vi "Pod Code.vi"() -> ()   [LabVIEW 2017]
uses:
  Type Defs/Relays.ctl
  Type Defs/tempReadings.ctl
  Sensors/Power Sensor - Adafruit INA219/INA219 Measurements.ctl
  Type Defs/telemetryReading.ctl
  <vilib>/Utility/RT CPU Load.ctl
  Type Defs/PodState.ctl
  Type Defs/tofReading.ctl
  Type Defs/pressureReading.ctl
  Type Defs/allLaserReadings.ctl
  Type Defs/laserReading.ctl
  Type Defs/AnalogPressureReading.ctl
  Type Defs/criticalTelemetry.ctl
  Sensors/Time of Flight - VL6180/VL6180 Resource.ctl
  Sensors/Power Sensor - Adafruit INA219/INA219 Config Options.ctl
  Type Defs/thermopileSettings.ctl
  Sensors/Pressure Sensor - BMP180/BMP180 Config Options.ctl
  Type Defs/SensorStates.ctl
  Type Defs/allData.ctl
  <vilib>/Platform/TimedLoop/XDataNode/timing_clust.ctl
  <vilib>/Platform/TimedLoop/XDataNode/nitl_modes.ctl
  <vilib>/Platform/TimedLoop/XDataNode/wakeup.ctl
  <vilib>/myRIO/Instrument Drivers/Onboard IO/DIO/typedefs/DIO Reference.ctl
  <vilib>/myRIO/Common/Instrument Driver Framework/Utilities/typedefs/myRIO Generic Hardware Reference.ctl
  <vilib>/myRIO/Common/Instrument Driver Framework/Utilities/typedefs/Hardware Version Enum.ctl
  <vilib>/myRIO/Common/Instrument Driver Framework/Utilities/typedefs/myRIO v1.0 Reference.ctl
  <vilib>/myRIO/Common/Instrument Driver Framework/Utilities/typedefs/Generic FPGA Reference.ctl
  <vilib>/myRIO/Common/Instrument Driver Framework/myRIO v1.0/DIO/typedefs/DIO Channels List.ctl
  <vilib>/myRIO/Common/Instrument Driver Framework/myRIO v1.0/DIO/typedefs/DIO Channels Enum.ctl
  <vilib>/userdefined/High Color/nirio_resource_hc.ctl
  <vilib>/myRIO/Common/Instrument Driver Framework/Utilities/vis/Is FPGA Ref Available.vi
  <vilib>/myRIO/Common/Instrument Driver Framework/myRIO v1.0/DIO/vis/myRIO v1.1 Open DIO.vi
  <vilib>/myRIO/Instrument Drivers/Onboard IO/DIO/vis/Read.vi
  <vilib>/myRIO/Instrument Drivers/Onboard IO/DIO/vis/Write.vi
  <vilib>/myRIO/Common/Instrument Driver Framework/Utilities/vis/Validate Channels.vi
  <vilib>/myRIO/Common/Instrument Driver Framework/myRIO v1.0/DIO/vis/myRIO v1.0 Reserve DIO.vi
  <vilib>/myRIO/Common/Instrument Driver Framework/myRIO v1.0/Resource Manager/vis/myRIO v1.0 Reserve Channel List.vi
  <vilib>/myRIO/Common/Instrument Driver Framework/myRIO v1.0/DIO/vis/myRIO v1.0 Build MUX Configuration DIO.vi
  <vilib>/myRIO/Common/Instrument Driver Framework/myRIO v1.0/Resource Manager/vis/myRIO v1.0 Reserve Channel.vi
  <vilib>/myRIO/Common/Instrument Driver Framework/myRIO v1.0/Resource Manager/vis/myRIO v1.0 Unreserve Channel.vi
  <vilib>/myRIO/Common/Instrument Driver Framework/myRIO v1.0/Resource Manager/vis/myRIO v1.0 Create Configuration List.vi
  <vilib>/myRIO/Common/Instrument Driver Framework/myRIO v1.0/Resource Manager/vis/myRIO v1.0 Build Mutex Name.vi
  <vilib>/Utility/VariantDataType/GetNumericInfo.vi
  <vilib>/Utility/error.llb/Error Cluster From Error Code.vi
  <vilib>/myRIO/Common/Instrument Driver Framework/myRIO v1.0/myRIO v1.1 Open.vi
  <vilib>/myRIO/Common/Instrument Driver Framework/Utilities/vis/IO Manager.vi
  <vilib>/myRIO/Common/Instrument Driver Framework/Utilities/vis/Configuration Manager.vi
  <vilib>/myRIO/Common/Instrument Driver Framework/myRIO v1.0/Resource Manager/vis/myRIO v1.0 Configure IO.vi
  <vilib>/myRIO/Common/Instrument Driver Framework/myRIO v1.0/myRIO v1.0 Close.vi
  <vilib>/myRIO/Common/Instrument Driver Framework/myRIO v1.0/DIO/vis/myRIO v1.0 Write DIO.vi
  <vilib>/myRIO/Common/Instrument Driver Framework/myRIO v1.0/DIO/vis/myRIO v1.0 Read DIO.vi
  <vilib>/myRIO/Express VI/Onboard IO/DO/DO Express VI.xnode
  <vilib>/myRIO/Instrument Drivers/Onboard IO/DIO/vis/myRIO DIO Open.xnode
  <vilib>/platform/TimedLoop/XDataNode/XDataNode.xnode
  <vilib>/myRIO/Express VI/Onboard IO/DI/DI Express VI.xnode
  <vilib>/myRIO/Instrument Drivers/Onboard IO/DIO/DIO.lvlib
  <vilib>/Platform/TimedLoop/XDataNode/XDNodeRunTimeDep.lvlib
  <vilib>/NI_Real-Time Target Support.lvlib
panel:
  in  "Prior Lows":u8=10
  out "Data Snap Period":u32
  out "Slow Sensor Period":u32
  out "State Machine Period":u32
  out "Fast Sensor Period":u32
  out "Actuators":u32
  out "Latest Critical Telemetry":T1
  out "Analog Pressure Reading":T3
  out "Laser Error":errorcluster
  out "Laser Readings":T4
  out "Pressure Reading":T6
  out "ToF Readings":T7[](array[typedef])
  out "Pod State Status":T2
  in  "Logging":bool
  out "Sensor Error 2":errorcluster
  out "# elements in queue":i32
  out "CPU loads":T8[](array[typedef]) {"ISR (%)" format="%#.2f"; "Idle (%)" format="%#.2f"; "Background (%)" format="%#.2f"; "Normal (%)" format="%#.2f"; "Above Normal (%)" format="%#.2f"; "High (%)" format="%#.2g"; "Timed Structures (%)" format="%#.2g"; "Time Critical (%)" format="%#.2g"; "Total (%)" format="%#.2g"}
  out "Log":T9[][](array[typedef])
  in  "Power I2C Addrs":u8[](array[numeric])=[68, 65, 69] format="%.0x"
  out "Power Readings":T10[](array[typedef]) {"Current" format="%#.3g A"; "Power" format="%#.3g W"; "Shunt Voltage" format=" %#.3g V"; "Bus Voltage" format="%#.3g V"; "Voltage (Total)" format="%#.3g V"}
  out "ThermalReadings":T11[](array[typedef]) {"Ambient Temp (°F)" format="%.2f °F"; "Ambient Temp (°C)" format="%.2f °C"; "Object Temp (°F)" format="%.2f °F"; "Object Temp (°C)" format="%.2f °C"}
  in  "Thermal I2C Addrs":u8[](array[numeric])=[64, 67] format="%.0x"
  in  "Reset Count":bool
  in  "ToFs in use":T12[](array[typedef])=[enum."ToF1", enum."ToF2", enum."ToF3", enum."ToF4"]
  out "Sensor Error":errorcluster
  in  "Reset Sensors":bool
  out "State Error":errorcluster
  in  "Stop Button":bool
  # "Config"
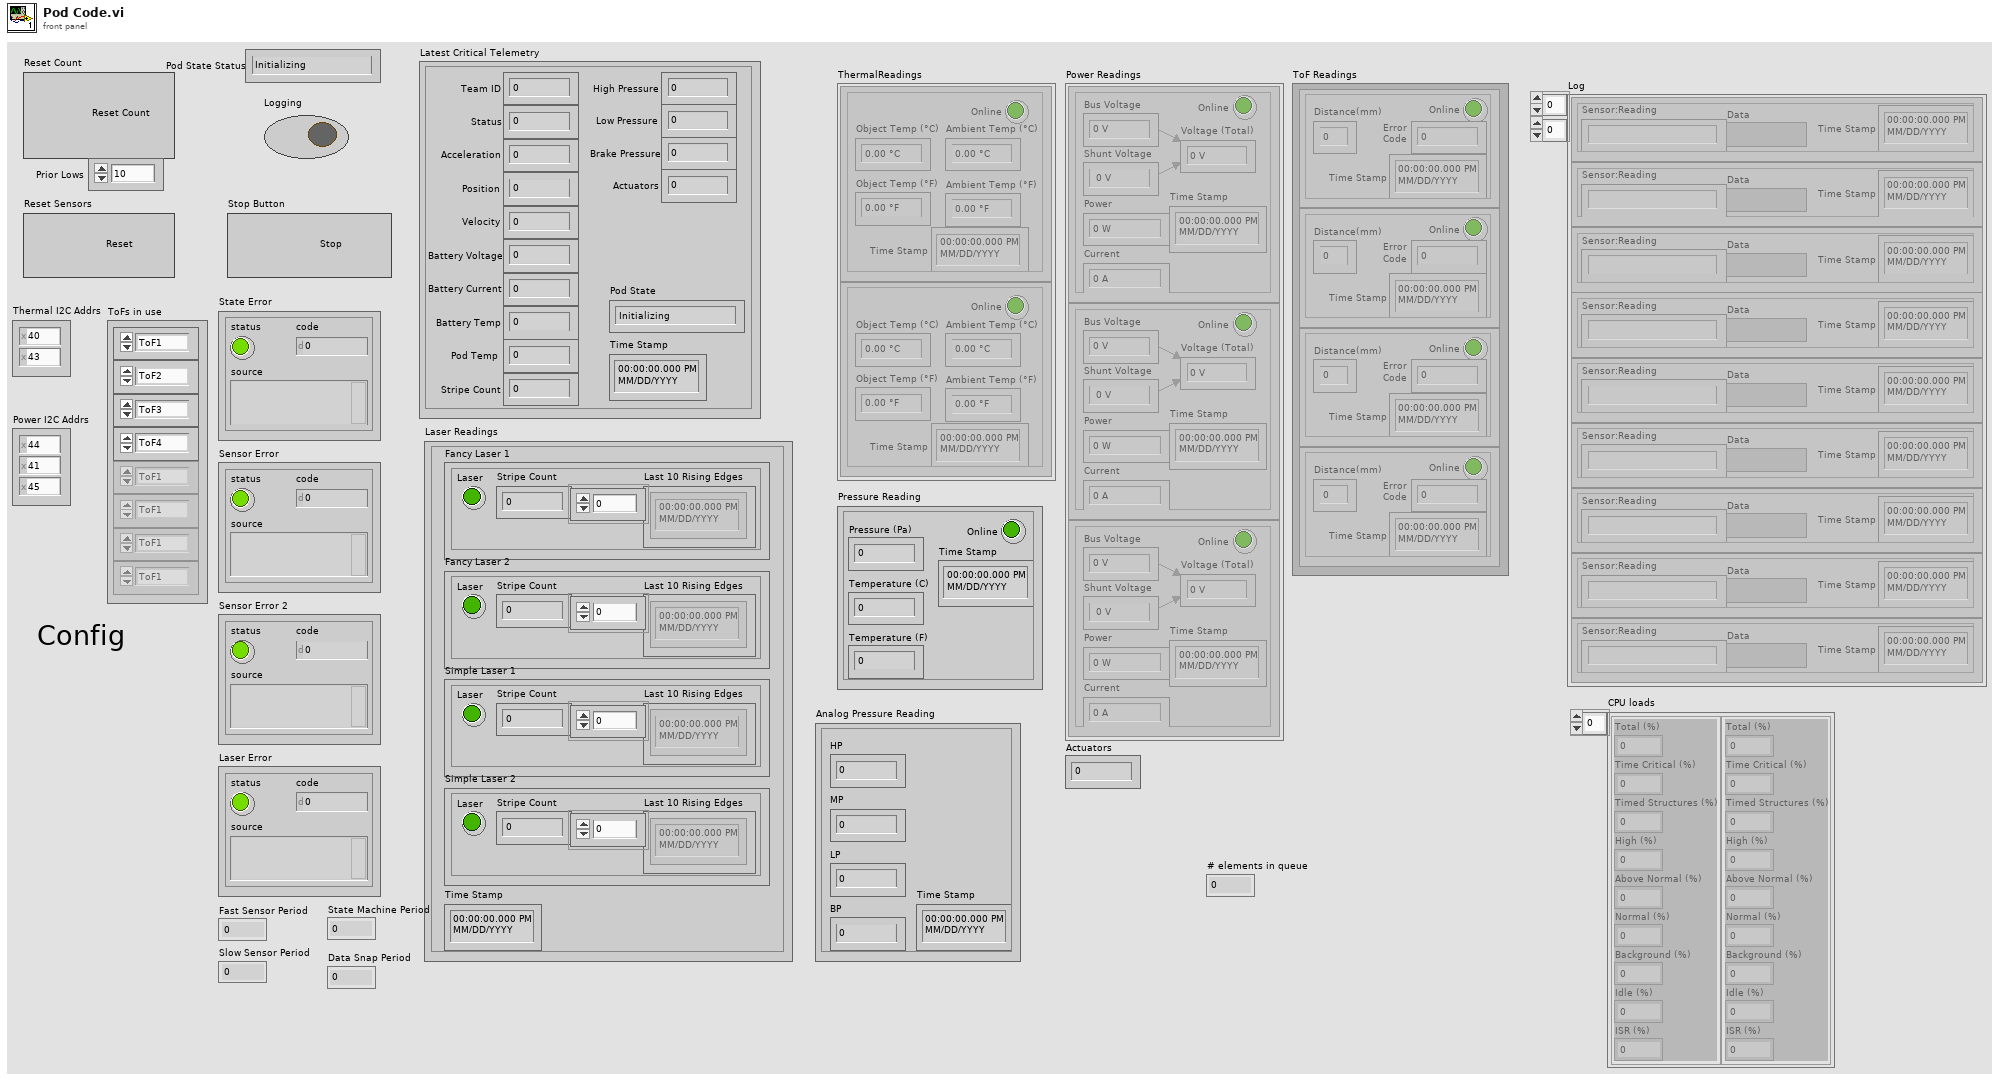
[diagram p1: front panel]
types:
  T1 = typedef "criticalTelemetry.ctl" = cluster{"Team ID":u8, "Status":u8, "Acceleration":i32, "Position":i32, "Velocity":i32, "Battery Voltage":i32, "Battery Current":i32, "Battery Temp":i32, "Pod Temp":i32, "Stripe Count":u32, "High Pressure":dbl, "Low Pressure":dbl, "Brake Pressure":dbl, "Actuators":u32, "Pod State":T2, "Time Stamp":timestamp}
  T2 = typedef "PodState.ctl" = enum16{"Initializing", "Pre-flight Testing", "Ready", "Pushing", "Coast", "Braking", "Post-flight", "Fault"}
  T3 = typedef "AnalogPressureReading.ctl" = cluster{"HP":dbl, "MP":dbl, "LP":dbl, "BP":dbl, "Time Stamp":timestamp}
  T4 = typedef "allLaserReadings.ctl" = cluster{"Fancy Laser 1":T5, "Fancy Laser 2":T5, "Simple Laser 1":T5, "Simple Laser 2":T5, "Time Stamp":timestamp}
  T5 = typedef "laserReading.ctl" = cluster{"Laser":bool, "Stripe Count":u32, "Last 10 Rising Edges":timestamp[]}
  T6 = typedef "pressureReading.ctl" = cluster{"Time Stamp":timestamp, "Online":bool, "Temperature (C)":dbl, "Pressure (Pa)":dbl, "Temperature (F)":dbl}
  T7 = typedef "tofReading.ctl" = cluster{"Distance(mm)":u8, "Online":bool, "Error\nCode":u8, "Time Stamp":timestamp}
  T8 = typedef "NI_Real-Time Target Support.lvlib/RT CPU Load.ctl" = cluster{"Total (%)":dbl, "Time Critical (%)":dbl, "Timed Structures (%)":dbl, "High (%)":dbl, "Above Normal (%)":dbl, "Normal (%)":dbl, "Background (%)":dbl, "Idle (%)":dbl, "ISR (%)":dbl}
  T9 = typedef "telemetryReading.ctl" = cluster{"Sensor:Reading":string, "Data":variant, "Time Stamp":timestamp}
  T10 = typedef "INA219 Measurements.ctl" = cluster{"Voltage (Total)":dbl, "Bus Voltage":dbl, "Shunt Voltage":dbl, "Power":dbl, "Current":dbl, "Online":bool, "Time Stamp":timestamp}
  T11 = typedef "tempReadings.ctl" = cluster{"Object Temp (°C)":dbl, "Object Temp (°F)":dbl, "Ambient Temp (°C)":dbl, "Ambient Temp (°F)":dbl, "Online":bool, "Time Stamp":timestamp}
  T12 = typedef "Relays.ctl" = enum16{"ToF1", "ToF2", "ToF3", "ToF4", "ToF5", "ToF6", "ToF7", "ToF8", "SensePwr", "All"}
  T13 = typedef "SensorStates.ctl" = enum16{"Reset", "Read", "Close"}
  T14 = typedef "BMP180 Config Options.ctl" = cluster{"I2C":cluster{"Slave Address":u8, "Channel":u8}, "Mode":enum8{"Ultra Low Power", "Standard", "High Resolution", "Ultra High Resolution"}, "Cal Coefs":cluster{"AC1":cluster{"Addr:":u8, "Val:":u16}, "AC2":cluster{"Addr:":u8, "Val:":u16}, "AC3":cluster{"Addr:":u8, "Val:":u16}, "AC4":cluster{"Addr:":u8, "Val:":u16}, "AC5":cluster{"Addr:":u8, "Val:":u16}, "AC6":cluster{"Addr:":u8, "Val:":u16}, "B1":cluster{"Addr:":u8, "Val:":u16}, "B2":cluster{"Addr:":u8, "Val:":u16}, "MB":cluster{"Addr:":u8, "Val:":u16}, "MC":cluster{"Addr:":u8, "Val:":u16}, "MD":cluster{"Addr:":u8, "Val:":u16}}, "Online":bool}
  T15 = typedef "thermopileSettings.ctl" = cluster{"Online":bool, "I2C Channel":u8, "I2C Slave Address":u8, "Valid Sample":bool, "Samples to Average":u16, "Last Temp Readings":T11, "Last Reading Time":dbl, "Last Conv Time":dbl}
  T16 = typedef "INA219 Config Options.ctl" = cluster{"I2C":cluster{"Slave Address":u8, "Channel":u8}, "Reset bit":u8, "Bus Voltage Range":u8, "PGA/Shunt Voltage Gain":u8, "Bus Voltage ADC Settings":u8, "Shunt Voltage ADC Settings":u8, "Mode":u8, "Calibration Value":u16, "Online":bool, "Shunt Resistor":dbl}
  T17 = typedef "VL6180 Resource.ctl" = cluster{"I2C Channel":u8, "I2C Slave Address":u8, "Online":bool}
  T18 = typedef "XDNodeRunTimeDep.lvlib/timing_clust.ctl" = cluster{"Expected End [f-1]":u64, "Actual End [f-1]":u64, "Finished Late? [f-1]":bool, "Expected End [i-1]":u64, "Actual End [i-1]":u64, "Finished Late? [i-1]":bool, "Expected Start [i]":u64, "Actual Start [i]":u64, "Expected Start [f]":u64, "Actual Start [f]":u64, "Source Name":string, "Structure Name":string, "Period":i64, "Deadline":i64, "Offset":i64, "Start":i64, "Priority":i32, "Timeout":i32, "Mode":T19, "Wakeup Reason":T20, "Error":errorcluster, "Source Type":string, "Secondary Source Type":string, "Global End Time":u64, "Global Start Time":u64, "Frame Duration":u64, "Iteration Duration":u64, "Assigned CPU":i32, "I/O Scan Engine Mode":u32}
  T19 = typedef "XDNodeRunTimeDep.lvlib/nitl_modes.ctl" = enum32{"No Change", "Process missed periods, maintain original phase", "Discard missed periods, maintain original phase", "Process missed periods, ignore original phase", "Discard missed periods, ignore original phase"}
  T20 = typedef "XDNodeRunTimeDep.lvlib/wakeup.ctl" = enum32{"Normal", "Aborted", "Asynchronous wakeup", "Timing source error", "Timed loop error", "Timeout"}
  T21 = typedef "DIO.lvlib/DIO Reference.ctl" = cluster{"myRIO Reference":T22, "DIO Channels List":T26}
  T22 = typedef "myRIO Generic Hardware Reference.ctl" = cluster{"myRIO Model":T23, "myRIO Hardware Reference":T24}
  T23 = typedef "Hardware Version Enum.ctl" = enum16{"Unknown", "myRIO-1900", "myRIO-1950", "roboRIO", "NI ELVIS RIO CM"}
  T24 = typedef "myRIO v1.0 Reference.ctl" = cluster{"Generic FPGA Reference":T25, "Allow multiple opens":bool}
  T25 = typedef "Generic FPGA Reference.ctl" = refnum<k20>
  T26 = typedef "DIO Channels List.ctl" = T27[]
  T27 = typedef "DIO Channels Enum.ctl" = enum16{"Not Connected", "C/DIO0", "C/DIO1", "C/DIO2", "C/DIO3", "C/DIO4", "C/DIO5", "C/DIO6", "C/DIO7", "A/DIO0", "A/DIO1", "A/DIO2", "A/DIO3", "A/DIO4", "A/DIO5", "A/DIO6", "A/DIO7", "A/DIO8", "A/DIO9", "A/DIO10", "A/DIO11", "A/DIO12", "A/DIO13", "A/DIO14", "A/DIO15", "B/DIO0", "B/DIO1", "B/DIO2", "B/DIO3", "B/DIO4", "B/DIO5", "B/DIO6", "B/DIO7", "B/DIO8", "B/DIO9", "B/DIO10", "B/DIO11", "B/DIO12", "B/DIO13", "B/DIO14", "B/DIO15", "LED0", "LED1", "LED2", "LED3", "Button0", "DIO/DIO0", "DIO/DIO1", "DIO/DIO2", "DIO/DIO3", "DIO/DIO4", "DIO/DIO5", "DIO/DIO6", "DIO/DIO7", "DIO/DIO8", "DIO/DIO9", "SPI/CS0", "SPI/CS1", "SPI/CS2", "SPI/CS3", "LED RADIO (Green)", "LED RADIO (Red)", "LED COMM (Green)", "LED COMM (Red)", "LED MODE (Green)", "LED MODE (Red)"}
  T28 = typedef "nirio_resource_hc.ctl" = tag
  T29 = typedef "allData.ctl" = cluster{"Power Readings":T10[], "ThermalReadings":T11[], "Analog Pressure Reading":T3, "Laser Readings":T4, "Pod State":T2, "seconds since 1Jan1904":timestamp, "ToF Readings":T7[], "CPU loads":T8[], "Actuators":u32, "Pressure Reading":T6, "Laser Error":errorcluster, "Sensor Error":errorcluster, "Sensor Error 2":errorcluster, "State Error":errorcluster}
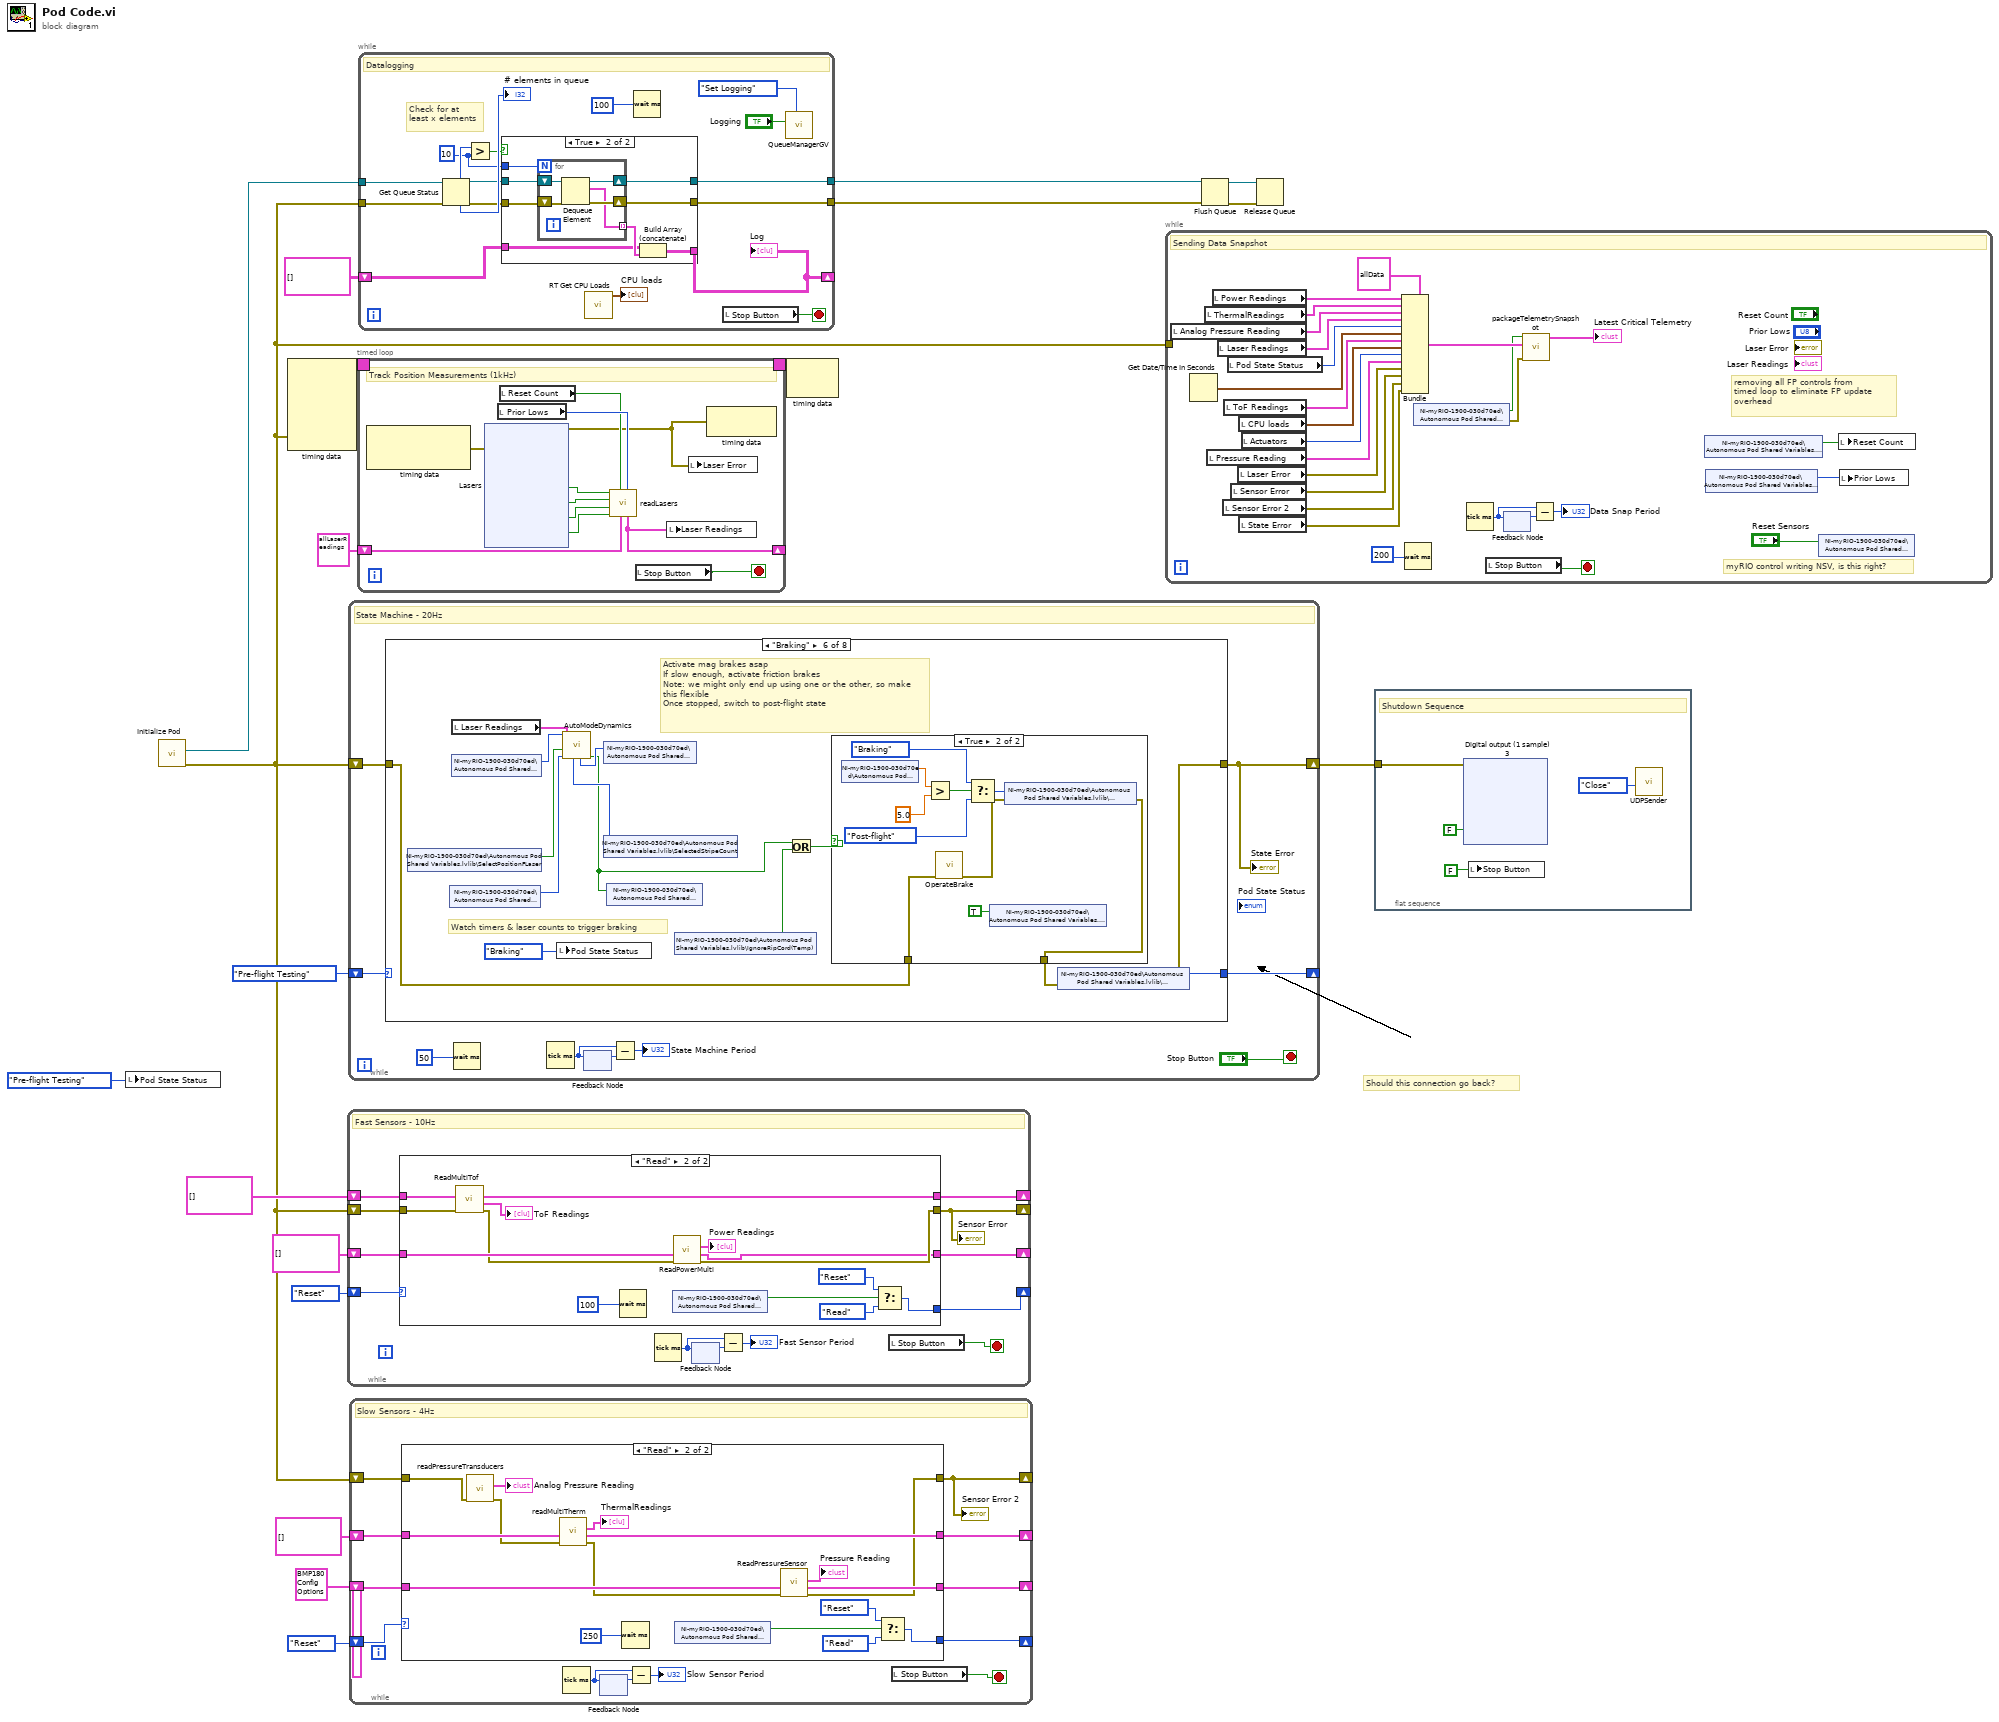
[diagram p0: block diagram]
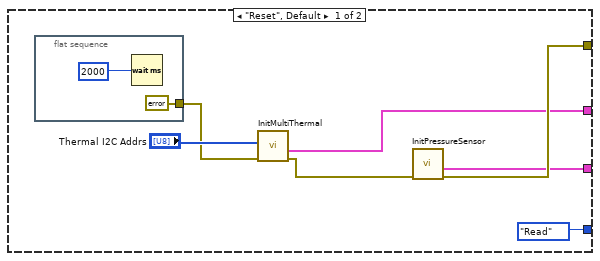
[diagram p3: hidden frame]
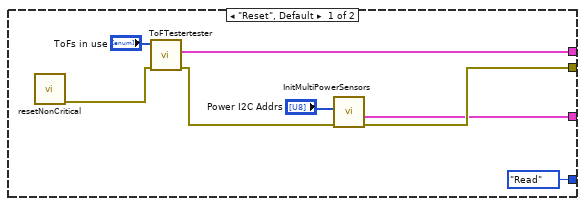
[diagram p4: hidden frame]
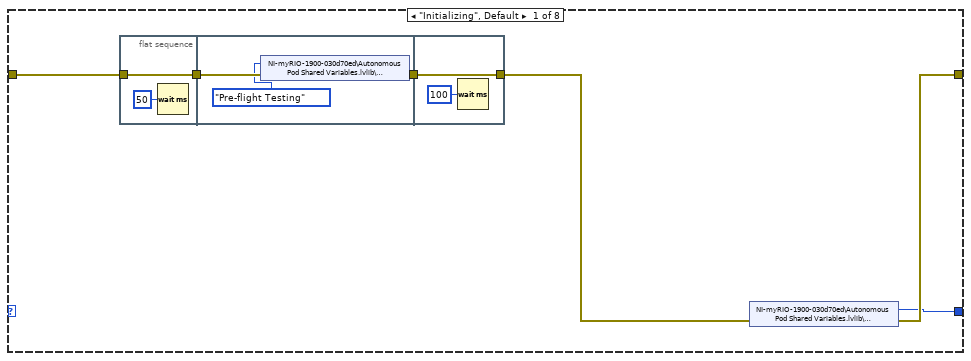
[diagram p5: hidden frame]
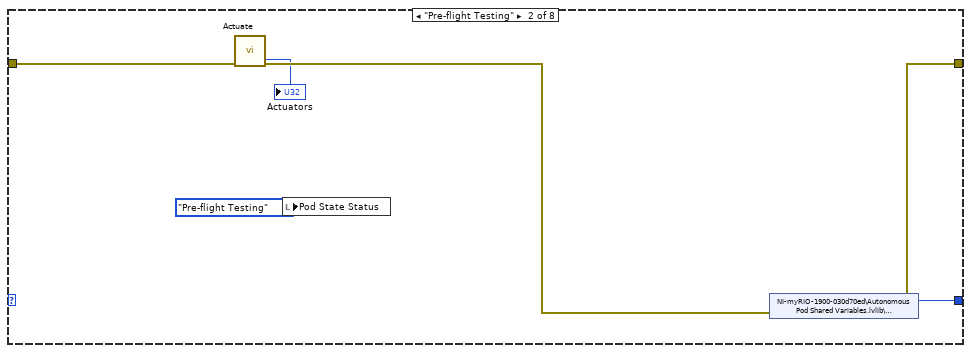
[diagram p6: hidden frame]
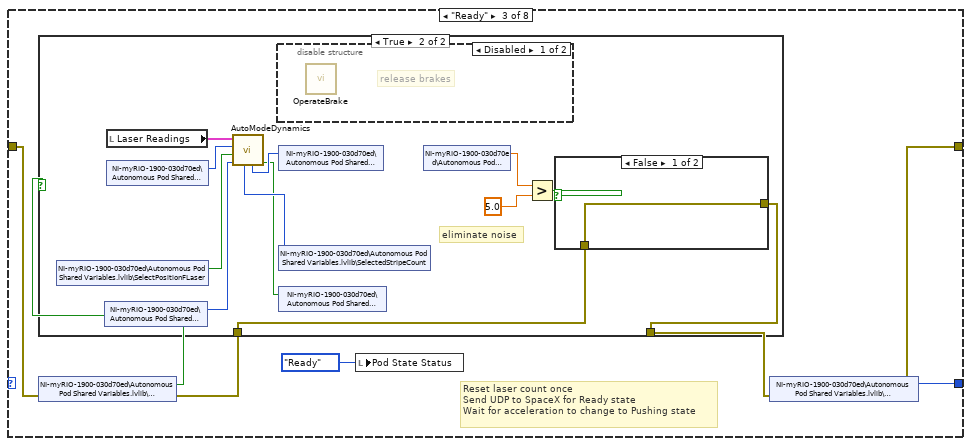
[diagram p7: hidden frame]
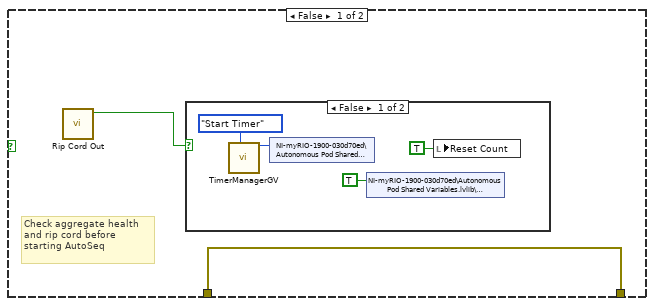
[diagram p8: hidden frame]
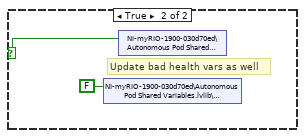
[diagram p9: hidden frame]
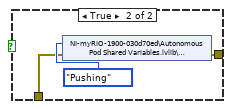
[diagram p11: hidden frame]
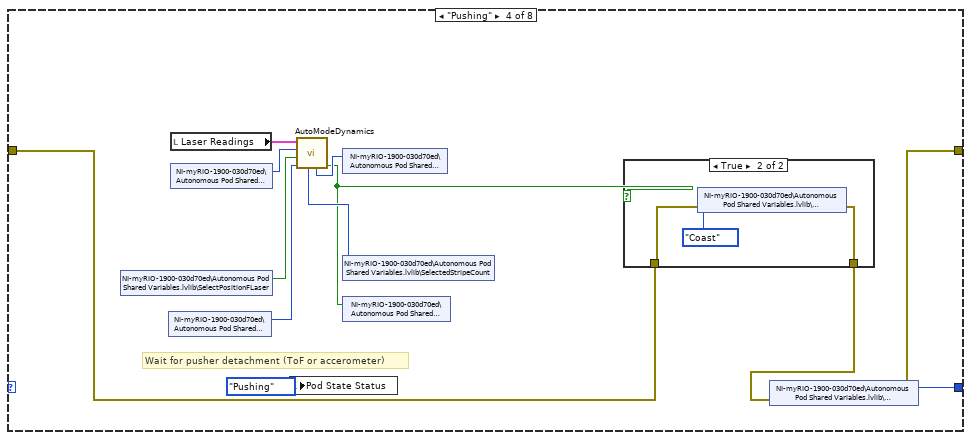
[diagram p12: hidden frame]
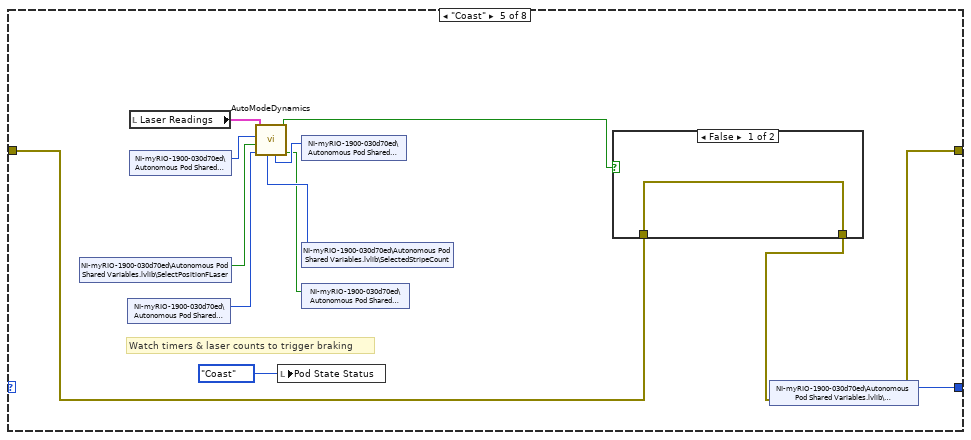
[diagram p14: hidden frame]
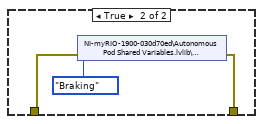
[diagram p15: hidden frame]
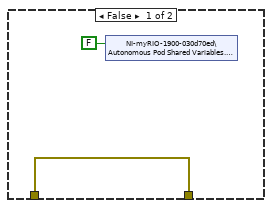
[diagram p16: hidden frame]
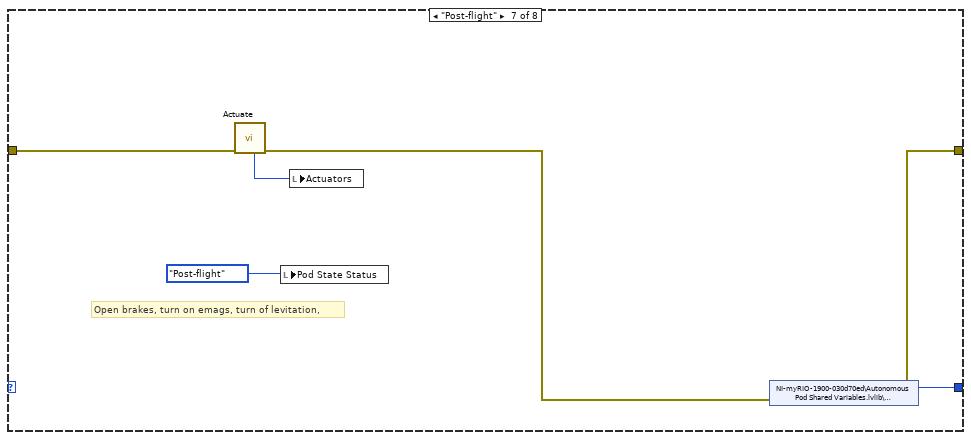
[diagram p17: hidden frame]
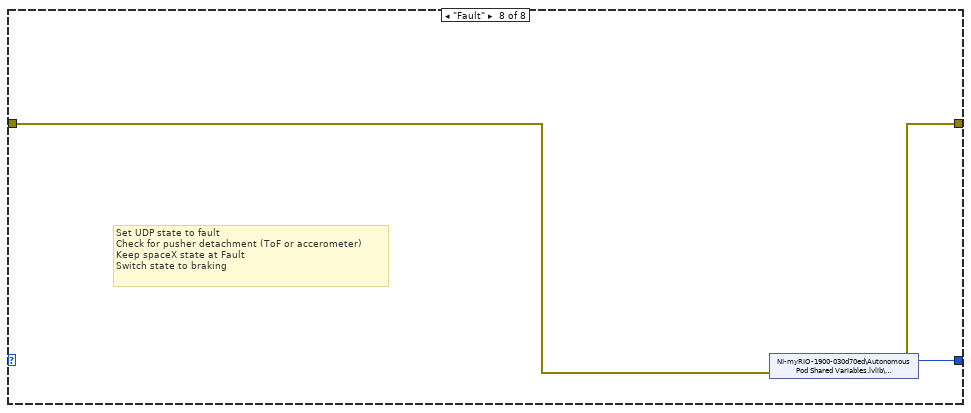
[diagram p18: hidden frame]
diagram:
  # "Should this connection go back?"
  n1 = local write "Pod State Status"(PodState."Pre-flight Testing" ("Pod State")) -> ()
  n2 = call "Initialize Pod.vi"() -> ("error out"=w3:errorcluster, "Telemetry Queue"=w16:refnum<queue>)  [unwired: 10 in]
  n3 = node-c288(w3) -> (w10:T18)  [unwired: 4 in]
  n4 = while {
    shift-right: [w29] -> _
    shift-left: SensorStates."Reset" -> [w31]
    shift-right: [w25] -> _
    shift-left: w3 -> [w30]
    shift-right: [w27] -> _
    shift-left: T17[] [] ("VL Configs") -> [w26]
    shift-right: [w20] -> _
    shift-left: T16[] [] ("Config Out") -> [w24]
    stop <- w28 stop-if-true
    # "Fast Sensors - 10Hz"
    n5 = case shown="\"Read\"" w31 {
      tunnel: w30 -> [_ w48]
      tunnel: [w35 w43] -> w25
      tunnel: [SensorStates."Read" w52] -> w29
      tunnel: [w32 w47] -> w27
      tunnel: w26 -> [_ w49]
      tunnel: w24 -> [_ w45]
      tunnel: [w33 w40] -> w20
      frame "Reset", Default {
        n6 = call "resetNonCritical.vi"() -> ("error out"=w38:errorcluster)  [unwired: 11 in]
        n7 = call "ToFTestertester.vi"("error in"=w38, "ToFs"="ToFs in use") -> ("error out"=w34:errorcluster, "ToF Details"=w32:T17[])  [unwired: 7 in, 1 out]
        n8 = call "InitMultiPowerSensors.vi"("error in"=w34, "I2C Addresses"="Power I2C Addrs") -> ("error out"=w35:errorcluster, "Power Sensors Configs"=w33:T16[])  [unwired: 7 in, 1 out]
      }
      frame "Read" {
        n9 = call "ReadMultiTof.vi"("error in"=w48, "VL6180 Resources"=w49) -> ("error out"=w42:errorcluster, "ToF Readings"=→"ToF Readings":T7[], "VL Configs"=w47:T17[])  [unwired: 6 in, 1 out]
        n10 = Wait (ms)(milliseconds to wait=u32 100) -> ()  [unwired: 1 out]
        n11 = shared-variable "NI-myRIO-1900-030d70ed\\Autonomous Pod Shared Variables.lvlib\\ResetSensor"() -> (w46:bool)  [unwired: 1 in, 1 out]
        n12 = call "ReadPowerMulti.vi"("error in"=w42, "Config In"=w45) -> ("error out"=w43:errorcluster, "Config Out"=w40:T16[], "Power Readings"=→"Power Readings":T10[])  [unwired: 7 in]
        n13 = Select(t=SensorStates."Reset", s=w46, f=SensorStates."Read") -> (s? t:f=w52:T13)
      }
    }
    "Sensor Error" <- w25
    n14 = Tick Count (ms)() -> (millisecond timer value=w22:u32)
    n15 = feedback-in #1(w22) -> ()
    n16 = feedback #1() -> (w23:u32)  [unwired: 1 in]
    n17 = Subtract(x=w22, y=w23) -> (x-y=→"Fast Sensor Period":u32)
    n18 = local read "Stop Button"() -> (w28:bool)
  }
  n19 = while {
    shift-right: [w58] -> w14
    shift-left: w3 -> [w60]
    shift-right: [w57] -> _
    shift-left: PodState."Pre-flight Testing" ("Pod States") -> [w59]
    stop <- "Stop Button" stop-if-true
    # "State Machine - 20Hz"
    n20 = case shown="\"Braking\"" w59 {
      tunnel: w60 -> [w68 w79 w85 w114 w131 w147 w175 w178]
      tunnel: [w64 w80 w87 w123 w140 w158 w176 w179] -> w58
      tunnel: [w63 w81 w88 w124 w141 w159 w177 w180] -> w57
      frame "Initializing", Default {
        n21 = flat-sequence {
          tunnel: w68 -> [w69]
          tunnel: [w69] -> w67
          tunnel: w67 -> [w73]
          tunnel: [w72] -> w65
          tunnel: [w74] -> w66
          tunnel: w65 -> [w74]
          frame #0 {
            n22 = Wait (ms)(milliseconds to wait=u32 50) -> ()  [unwired: 1 out]
          }
          frame #1 {
            n23 = shared-variable "NI-myRIO-1900-030d70ed\\Autonomous Pod Shared Variables.lvlib\\PodStateCommand"(PodState."Pre-flight Testing" ("Pod States"), error in=w73) -> (error out=w72:errorcluster)
          }
          frame #2 {
            n24 = Wait (ms)(milliseconds to wait=u32 100) -> ()  [unwired: 1 out]
          }
        }
        n25 = shared-variable "NI-myRIO-1900-030d70ed\\Autonomous Pod Shared Variables.lvlib\\PodStateCommand"(error in=w66) -> (w63:T2, error out=w64:errorcluster)
      }
      frame "Pre-flight Testing" {
        n26 = call "Actuate.vi"("error in"=w79) -> ("error out"=w78:errorcluster, "Actuators"=→"Actuators":u32)  [unwired: 8 in, 1 out]
        n27 = local write "Pod State Status"(PodState."Pre-flight Testing" ("Pod State")) -> ()
        n28 = shared-variable "NI-myRIO-1900-030d70ed\\Autonomous Pod Shared Variables.lvlib\\PodStateCommand"(error in=w78) -> (w81:T2, error out=w80:errorcluster)
      }
      frame "Ready" {
        # "Reset laser count once\nSend UDP to SpaceX for Ready state\nWait for acceleration to change to Pushing state"
        n29 = shared-variable "NI-myRIO-1900-030d70ed\\Autonomous Pod Shared Variables.lvlib\\AutoSequenceOn"(error in=w85) -> (w86:bool, error out=w83:errorcluster)
        n30 = case shown="True" w86 {
          tunnel: w83 -> [w89 w98]
          tunnel: [w89 w97] -> w82
          frame False {
            # "Check aggregate health and rip cord before starting AutoSeq"
            n31 = call "Rip Cord Out"() -> ("Rip Cord Out?"=w90:bool)  [unwired: 11 in]
            n32 = case shown="False" w90 {
              selector: w90 -> [_ w96]
              frame False {
                n33 = call "TimerManagerGV.vi"("Command"=enum16{"Get Time Elapsed", "Start Timer"}."Start Timer") -> ("Timer Value(s)"=w91:u32)  [unwired: 9 in, 1 out]
                n34 = shared-variable "NI-myRIO-1900-030d70ed\\Autonomous Pod Shared Variables.lvlib\\TimerValue"(w91) -> ()  [unwired: 1 in, 1 out]
                n35 = shared-variable "NI-myRIO-1900-030d70ed\\Autonomous Pod Shared Variables.lvlib\\AutoSequenceOn"(TRUE ("AutoSequenceOn")) -> ()  [unwired: 1 in, 1 out]
                n36 = local write "Reset Count"(TRUE ("Reset Count")) -> ()
              }
              frame True {
                # "Update bad health vars as well"
                n37 = shared-variable "NI-myRIO-1900-030d70ed\\Autonomous Pod Shared Variables.lvlib\\AutoSequenceOn"(FALSE ("AutoSequenceOn")) -> ()  [unwired: 1 in, 1 out]
                n38 = shared-variable "NI-myRIO-1900-030d70ed\\Autonomous Pod Shared Variables.lvlib\\RipCordOut"(w96) -> ()  [unwired: 1 in, 1 out]
              }
            }
          }
          frame True {
            # "eliminate noise"
            n39 = shared-variable "NI-myRIO-1900-030d70ed\\Autonomous Pod Shared Variables.lvlib\\SelectPositionFLaser"() -> (w106:bool)  [unwired: 1 in, 1 out]
            n40 = shared-variable "NI-myRIO-1900-030d70ed\\Autonomous Pod Shared Variables.lvlib\\TimerLimit"() -> (w105:u32)  [unwired: 1 in, 1 out]
            n41 = local read "Laser Readings"() -> (w107:T4)
            n42 = shared-variable "NI-myRIO-1900-030d70ed\\Autonomous Pod Shared Variables.lvlib\\StripeLimit"() -> (w108:u32)  [unwired: 1 in, 1 out]
            n43 = call "AutoModeDynamics.vi"("Timer Limit"=w105, "SelectFLaser"=w106, "Stripe Limit"=w108, "Laser Readings"=w107) -> ("Rip Cord Out?"=w102:bool, "Timer Value(s)"=w104:u32, "Stripe Count"=w103:u32)  [unwired: 2 in, 3 out]
            n44 = disable-structure shown="Disabled" {
              frame Disabled {
                # "release brakes"
                n45 = call "OperateBrake.vi"() -> ()  [unwired: 11 in, 1 out]
              }
              frame Enabled {
              }
            }
            n46 = shared-variable "NI-myRIO-1900-030d70ed\\Autonomous Pod Shared Variables.lvlib\\TimerValue"(w104) -> ()  [unwired: 1 in, 1 out]
            n47 = shared-variable "NI-myRIO-1900-030d70ed\\Autonomous Pod Shared Variables.lvlib\\SelectedStripeCount"(w103) -> ()  [unwired: 1 in, 1 out]
            n48 = shared-variable "NI-myRIO-1900-030d70ed\\Autonomous Pod Shared Variables.lvlib\\RipCordOut"(w102) -> ()  [unwired: 1 in, 1 out]
            n49 = shared-variable "NI-myRIO-1900-030d70ed\\Autonomous Pod Shared Variables.lvlib\\Velocity"() -> (w101:dbl)  [unwired: 1 in, 1 out]
            n50 = Greater?(x=w101, y=5.0) -> (0:w99:bool)
            n51 = case shown="False" w99 {
              tunnel: w98 -> [w109 w111]
              tunnel: [w109 w110] -> w97
              frame False {
              }
              frame True {
                n52 = shared-variable "NI-myRIO-1900-030d70ed\\Autonomous Pod Shared Variables.lvlib\\PodStateCommand"(PodState."Pushing" ("Pod States"), error in=w111) -> (error out=w110:errorcluster)
              }
            }
          }
        }
        n53 = local write "Pod State Status"(PodState."Ready" ("Pod State")) -> ()
        n54 = shared-variable "NI-myRIO-1900-030d70ed\\Autonomous Pod Shared Variables.lvlib\\PodStateCommand"(error in=w82) -> (w88:T2, error out=w87:errorcluster)
      }
      frame "Pushing" {
        # "Wait for pusher detachment (ToF or accerometer)"
        n55 = shared-variable "NI-myRIO-1900-030d70ed\\Autonomous Pod Shared Variables.lvlib\\SelectPositionFLaser"() -> (w119:bool)  [unwired: 1 in, 1 out]
        n56 = shared-variable "NI-myRIO-1900-030d70ed\\Autonomous Pod Shared Variables.lvlib\\TimerLimit"() -> (w118:u32)  [unwired: 1 in, 1 out]
        n57 = local read "Laser Readings"() -> (w120:T4)
        n58 = shared-variable "NI-myRIO-1900-030d70ed\\Autonomous Pod Shared Variables.lvlib\\StripeLimit"() -> (w121:u32)  [unwired: 1 in, 1 out]
        n59 = local write "Pod State Status"(PodState."Pushing" ("Pod State")) -> ()
        n60 = call "AutoModeDynamics.vi"("Timer Limit"=w118, "SelectFLaser"=w119, "Stripe Limit"=w121, "Laser Readings"=w120) -> ("Rip Cord Out?"=w115:bool, "Timer Value(s)"=w117:u32, "Stripe Count"=w116:u32)  [unwired: 2 in, 3 out]
        n61 = shared-variable "NI-myRIO-1900-030d70ed\\Autonomous Pod Shared Variables.lvlib\\TimerValue"(w117) -> ()  [unwired: 1 in, 1 out]
        n62 = shared-variable "NI-myRIO-1900-030d70ed\\Autonomous Pod Shared Variables.lvlib\\SelectedStripeCount"(w116) -> ()  [unwired: 1 in, 1 out]
        n63 = shared-variable "NI-myRIO-1900-030d70ed\\Autonomous Pod Shared Variables.lvlib\\RipCordOut"(w115) -> ()  [unwired: 1 in, 1 out]
        n64 = case shown="True" w115 {
          tunnel: w114 -> [w125 w127]
          tunnel: [w125 w126] -> w113
          frame False {
          }
          frame True {
            n65 = shared-variable "NI-myRIO-1900-030d70ed\\Autonomous Pod Shared Variables.lvlib\\PodStateCommand"(PodState."Coast" ("PodStateCommand"), error in=w127) -> (error out=w126:errorcluster)
          }
        }
        n66 = shared-variable "NI-myRIO-1900-030d70ed\\Autonomous Pod Shared Variables.lvlib\\PodStateCommand"(error in=w113) -> (w124:T2, error out=w123:errorcluster)
      }
      frame "Coast" {
        # "Watch timers & laser counts to trigger braking"
        n67 = shared-variable "NI-myRIO-1900-030d70ed\\Autonomous Pod Shared Variables.lvlib\\SelectPositionFLaser"() -> (w137:bool)  [unwired: 1 in, 1 out]
        n68 = shared-variable "NI-myRIO-1900-030d70ed\\Autonomous Pod Shared Variables.lvlib\\TimerLimit"() -> (w136:u32)  [unwired: 1 in, 1 out]
        n69 = local read "Laser Readings"() -> (w138:T4)
        n70 = shared-variable "NI-myRIO-1900-030d70ed\\Autonomous Pod Shared Variables.lvlib\\StripeLimit"() -> (w139:u32)  [unwired: 1 in, 1 out]
        n71 = call "AutoModeDynamics.vi"("Timer Limit"=w136, "SelectFLaser"=w137, "Stripe Limit"=w139, "Laser Readings"=w138) -> ("Rip Cord Out?"=w133:bool, "Brake Condition Reached?"=w129:bool, "Timer Value(s)"=w135:u32, "Stripe Count"=w134:u32)  [unwired: 2 in, 2 out]
        n72 = local write "Pod State Status"(PodState."Coast" ("Pod State")) -> ()
        n73 = shared-variable "NI-myRIO-1900-030d70ed\\Autonomous Pod Shared Variables.lvlib\\TimerValue"(w135) -> ()  [unwired: 1 in, 1 out]
        n74 = shared-variable "NI-myRIO-1900-030d70ed\\Autonomous Pod Shared Variables.lvlib\\SelectedStripeCount"(w134) -> ()  [unwired: 1 in, 1 out]
        n75 = shared-variable "NI-myRIO-1900-030d70ed\\Autonomous Pod Shared Variables.lvlib\\RipCordOut"(w133) -> ()  [unwired: 1 in, 1 out]
        n76 = case shown="False" w129 {
          tunnel: w131 -> [w142 w144]
          tunnel: [w142 w143] -> w130
          frame False {
          }
          frame True {
            n77 = shared-variable "NI-myRIO-1900-030d70ed\\Autonomous Pod Shared Variables.lvlib\\PodStateCommand"(PodState."Braking" ("PodStateCommand"), error in=w144) -> (error out=w143:errorcluster)
          }
        }
        n78 = shared-variable "NI-myRIO-1900-030d70ed\\Autonomous Pod Shared Variables.lvlib\\PodStateCommand"(error in=w130) -> (w141:T2, error out=w140:errorcluster)
      }
      frame "Braking" {
        # "Watch timers & laser counts to trigger braking"
        # "Activate mag brakes asap\nIf slow enough, activate friction brakes\nNote: we might only end up using one or the other, so make this flexible\nOnce stopped, switch to post-flight state"
        n79 = shared-variable "NI-myRIO-1900-030d70ed\\Autonomous Pod Shared Variables.lvlib\\SelectPositionFLaser"() -> (w155:bool)  [unwired: 1 in, 1 out]
        n80 = shared-variable "NI-myRIO-1900-030d70ed\\Autonomous Pod Shared Variables.lvlib\\TimerLimit"() -> (w154:u32)  [unwired: 1 in, 1 out]
        n81 = local read "Laser Readings"() -> (w156:T4)
        n82 = shared-variable "NI-myRIO-1900-030d70ed\\Autonomous Pod Shared Variables.lvlib\\StripeLimit"() -> (w157:u32)  [unwired: 1 in, 1 out]
        n83 = local write "Pod State Status"(PodState."Braking" ("Pod State")) -> ()
        n84 = call "AutoModeDynamics.vi"("Timer Limit"=w154, "SelectFLaser"=w155, "Stripe Limit"=w157, "Laser Readings"=w156) -> ("Rip Cord Out?"=w149:bool, "Timer Value(s)"=w153:u32, "Stripe Count"=w152:u32)  [unwired: 2 in, 3 out]
        n85 = shared-variable "NI-myRIO-1900-030d70ed\\Autonomous Pod Shared Variables.lvlib\\TimerValue"(w153) -> ()  [unwired: 1 in, 1 out]
        n86 = shared-variable "NI-myRIO-1900-030d70ed\\Autonomous Pod Shared Variables.lvlib\\SelectedStripeCount"(w152) -> ()  [unwired: 1 in, 1 out]
        n87 = shared-variable "NI-myRIO-1900-030d70ed\\Autonomous Pod Shared Variables.lvlib\\RipCordOut"(w149) -> ()  [unwired: 1 in, 1 out]
        n88 = shared-variable "NI-myRIO-1900-030d70ed\\Autonomous Pod Shared Variables.lvlib\\IgnoreRipCord(Temp)"() -> (w148:bool)  [unwired: 1 in, 1 out]
        n89 = Or(x=w149, y=w148) -> (x .or. y?=w150:bool)
        n90 = case shown="True" w150 {
          tunnel: [w161 w171] -> w146
          tunnel: w147 -> [w161 w163]
          frame False {
            n91 = shared-variable "NI-myRIO-1900-030d70ed\\Autonomous Pod Shared Variables.lvlib\\OperatingBrakes"(FALSE ("OperatingBrakes")) -> ()  [unwired: 1 in, 1 out]
          }
          frame True {
            n92 = shared-variable "NI-myRIO-1900-030d70ed\\Autonomous Pod Shared Variables.lvlib\\Velocity"() -> (w170:dbl)  [unwired: 1 in, 1 out]
            n93 = Greater?(x=w170, y=5.0) -> (0:w168:bool)
            n94 = call "OperateBrake.vi"("error in"=w163) -> ("error out"=w164:errorcluster)  [unwired: 10 in]
            n95 = Select(t=PodState."Braking" ("PodStateCommand"), s=w168, f=PodState."Post-flight" ("PodStateCommand")) -> (s? t:f=w166:T2)
            n96 = shared-variable "NI-myRIO-1900-030d70ed\\Autonomous Pod Shared Variables.lvlib\\OperatingBrakes"(TRUE ("OperatingBrakes")) -> ()  [unwired: 1 in, 1 out]
            n97 = shared-variable "NI-myRIO-1900-030d70ed\\Autonomous Pod Shared Variables.lvlib\\PodStateCommand"(w166, error in=w164) -> (error out=w171:errorcluster)
          }
        }
        n98 = shared-variable "NI-myRIO-1900-030d70ed\\Autonomous Pod Shared Variables.lvlib\\PodStateCommand"(error in=w146) -> (w159:T2, error out=w158:errorcluster)
      }
      frame "Post-flight" {
        # "Open brakes, turn on emags, turn of levitation,"
        n99 = call "Actuate.vi"("error in"=w175) -> ("error out"=w174:errorcluster, "Actuators"=w173:u32)  [unwired: 8 in, 1 out]
        n100 = local write "Pod State Status"(PodState."Post-flight" ("Pod State")) -> ()
        n101 = local write "Actuators"(w173) -> ()
        n102 = shared-variable "NI-myRIO-1900-030d70ed\\Autonomous Pod Shared Variables.lvlib\\PodStateCommand"(error in=w174) -> (w177:T2, error out=w176:errorcluster)
      }
      frame "Fault" {
        # "Set UDP state to fault\nCheck for pusher detachment (ToF or accerometer)\nKeep spaceX state at Fault\nSwitch state to braking"
        n103 = shared-variable "NI-myRIO-1900-030d70ed\\Autonomous Pod Shared Variables.lvlib\\PodStateCommand"(error in=w178) -> (w180:T2, error out=w179:errorcluster)
      }
    }
    "State Error" <- w58
    n104 = Wait (ms)(milliseconds to wait=u32 50) -> ()  [unwired: 1 out]
    n105 = Tick Count (ms)() -> (millisecond timer value=w54:u32)
    n106 = feedback #2() -> (w55:u32)  [unwired: 1 in]
    n107 = feedback-in #2(w54) -> ()
    n108 = Subtract(x=w54, y=w55) -> (x-y=→"State Machine Period":u32)
  }
  n109 = while {
    shift-right: [w190] -> _
    shift-left: SensorStates."Reset" -> [w192]
    shift-right: [w188] -> _
    shift-left: w3 -> [w191]
    shift-right: [w187] -> _
    shift-left: T15[] [] ("ThermalConfigs") -> [w186]
    shift-right: [w185] -> _
    shift-left: T14 {"I2C"={"Slave Address"=64, "Channel"=0}, "Mode"=enum."Ultra Low Power", "Cal Coefs"={"AC1"={"Addr:"=170, "Val:"=0}, "AC2"={"Addr:"=172, "Val:"=0}, "AC3"={"Addr:"=174, "Val:"=0}, "AC4"={"Addr:"=176, "Val:"=0}, "AC5"={"Addr:"=178, "Val:"=0}, "AC6"={"Addr:"=180, "Val:"=0}, "B1"={"Addr:"=182, "Val:"=0}, "B2"={"Addr:"=184, "Val:"=0}, "MB"={"Addr:"=186, "Val:"=0}, "MC"={"Addr:"=188, "Val:"=0}, "MD"={"Addr:"=190, "Val:"=0}}, "Online"=FALSE} ("BMP180 Config Options") -> [w184]
    stop <- w189 stop-if-true
    # "Slow Sensors - 4Hz"
    n110 = case shown="\"Read\"" w192 {
      tunnel: w191 -> [_ w205]
      tunnel: [w198 w208] -> w188
      tunnel: [SensorStates."Read" w216] -> w190
      tunnel: [w193 w212] -> w187
      tunnel: w186 -> [_ w211]
      tunnel: [w195 w209] -> w185
      tunnel: w184 -> [_ w210]
      frame "Reset", Default {
        n111 = flat-sequence {
          tunnel: [errorcluster {"status"=FALSE, "code"=0, "source"=""} ("error in")] -> w194
          frame #0 {
            n112 = Wait (ms)(milliseconds to wait=u32 2000) -> ()  [unwired: 1 out]
          }
        }
        n113 = call "InitMultiThermal.vi"("error in"=w194, "I2C Addresses"="Thermal I2C Addrs") -> ("error out"=w196:errorcluster, "ThermalConfigs"=w193:T15[])  [unwired: 6 in, 2 out]
        n114 = call "InitPressureSensor.vi"("error in"=w196) -> ("error out"=w198:errorcluster, "BMP180 Config Options"=w195:T14)  [unwired: 9 in]
      }
      frame "Read" {
        n115 = call "readPressureTransducers.vi"("error in"=w205) -> ("error out"=w204:errorcluster, "Analog Pressure Reading"=→"Analog Pressure Reading":T3)  [unwired: 9 in]
        n116 = call "readMultiTherm.vi"("error in"=w204, "ThermalConfigs"=w211) -> ("error out"=w206:errorcluster, "ThermalConfigs"=w212:T15[], "ThermReadings"=→"ThermalReadings":T11[])  [unwired: 6 in, 1 out]
        n117 = Wait (ms)(milliseconds to wait=u32 250) -> ()  [unwired: 1 out]
        n118 = shared-variable "NI-myRIO-1900-030d70ed\\Autonomous Pod Shared Variables.lvlib\\ResetSensor"() -> (w213:bool)  [unwired: 1 in, 1 out]
        n119 = call "ReadPressureSensor.vi"("error in (no error)"=w206, "BMP180 Config Options"=w210) -> ("error out"=w208:errorcluster, "BMP180 Config"=w209:T14, "Pressure Reading"=→"Pressure Reading":T6)  [unwired: 7 in]
        n120 = Select(t=SensorStates."Reset", s=w213, f=SensorStates."Read") -> (s? t:f=w216:T13)
      }
    }
    "Sensor Error 2" <- w188
    n121 = Tick Count (ms)() -> (millisecond timer value=w181:u32)
    n122 = feedback #3() -> (w183:u32)  [unwired: 1 in]
    n123 = feedback-in #3(w181) -> ()
    n124 = Subtract(x=w181, y=w183) -> (x-y=→"Slow Sensor Period":u32)
    n125 = local read "Stop Button"() -> (w189:bool)
  }
  n126 = timed-loop {
    timing: w10 -> [_]
    timing-out: [_] -> w9
    shift-right: [w218] -> _
    shift-left: T4 {"Fancy Laser 1"={"Laser"=FALSE, "Stripe Count"=0, "Last 10 Rising Edges"=[]}, "Fancy Laser 2"={"Laser"=FALSE, "Stripe Count"=0, "Last 10 Rising Edges"=[]}, "Simple Laser 1"={"Laser"=FALSE, "Stripe Count"=0, "Last 10 Rising Edges"=[]}, "Simple Laser 2"={"Laser"=FALSE, "Stripe Count"=0, "Last 10 Rising Edges"=[]}, "Time Stamp"=timestamp(0 s since 1904-01-01)} ("Laser Readings") -> [w222]
    stop <- w228 stop-if-true
    # "Track Position Measurements (1kHz)"
    n127 = node-c288() -> (w227:errorcluster)  [unwired: 1 in, 1 out]
    n128 = xnode "Lasers"("error in (no error)"=w227) -> ("Fancy Laser 1 (B/DIO11 (Pin 18))"=w225:bool, "Fancy Laser 2 (A/DIO7 (Pin 25))"=w223:bool, "Laser 1 (B/DIO9 (Pin 29))"=w226:bool, "Laser 2 (B/DIO10 (Pin 31))"=w224:bool, "error out"=w219:errorcluster)
    n129 = local read "Prior Lows"() -> (w221:u8)
    n130 = local read "Reset Count"() -> (w220:bool)
    n131 = call "readLasers.vi"("Prior Lows"=w221, "Laser Readings In"=w222, "Reset Count"=w220, "Simple Laser 2"=w224, "Simple Laser 1"=w226, "Fancy Laser 2"=w223, "Fancy Laser 1"=w225) -> ("Laser Readings"=w218:T4)  [unwired: 4 in]
    n132 = local read "Stop Button"() -> (w228:bool)
    n133 = local write "Laser Readings"(w218) -> ()
    n134 = local write "Laser Error"(w219) -> ()
    n135 = node-c288(w219) -> ()  [unwired: 1 out]
  }
  n136 = while {
    tunnel: w3 -> [w286]
    tunnel: w16 -> [w284]
    tunnel: [w279] -> w6
    tunnel: [w278] -> w5
    shift-right: [w277] -> _
    shift-left: T9[][] [] -> [w276]
    stop <- w287 stop-if-true
    w282 = 10 ("y")
    # "Check for at least x elements"
    # "Datalogging"
    n137 = Get Queue Status(queue=w284, error in (no error)=w286) -> (queue out=w281:refnum<queue>, error out=w280:errorcluster, # elements in queue=w285:i32)  [unwired: 1 in, 5 out]
    "# elements in queue" <- w285
    n138 = Greater?(x=w285, y=w282) -> (0:w283:bool)
    n139 = case shown="True" w283 {
      tunnel: w282 -> [_ w298]
      tunnel: w281 -> [w290 w297]
      tunnel: w280 -> [w289 w296]
      tunnel: [w290 w295] -> w279
      tunnel: [w289 w294] -> w278
      tunnel: [w288 w291] -> w277
      tunnel: w276 -> [w288 w292]
      frame False {
      }
      frame True {
        n140 = for {
          N: w298 -> [_]
          shift-right: [w301] -> w295
          shift-left: w297 -> [w303]
          shift-right: [w300] -> w294
          shift-left: w296 -> [w302]
          tunnel: [w299] -> w293 mode=indexing
          n141 = Dequeue Element(queue=w303, error in (no error)=w302) -> (queue out=w301:refnum<queue>, element=w299:T9, error out=w300:errorcluster)  [unwired: 1 in, 1 out]
        }
        n142 = Build Array (concatenate)(w292, w293) -> (w291:T9[][])
      }
    }
    "Log" <- w277
    n143 = call <vilib>:"RT Get CPU Loads.vi"() -> ("CPU loads"=→"CPU loads":T8[])  [unwired: 10 in, 1 out]
    n144 = Wait (ms)(milliseconds to wait=u32 100) -> ()  [unwired: 1 out]
    n145 = local read "Stop Button"() -> (w287:bool)
    n146 = call "QueueManagerGV.vi"("Command"=enum16{"Get", "Set Logging", "Set Queue"}."Set Logging", "Logging"="Logging") -> ()  [unwired: 8 in, 2 out]
  }
  n147 = node-c288(w9) -> ()  [unwired: 1 out]
  n148 = while {
    tunnel: w3 -> [_]
    stop <- w330 stop-if-true
    # "myRIO control writing NSV, is this right?"
    # "removing all FP controls from \ntimed loop to eliminate FP update \noverhead"
    # "Sending Data Snapshot"
    n149 = local read "Analog Pressure Reading"() -> (w326:T3)
    n150 = Get Date/Time In Seconds() -> (seconds since 1Jan1904=w323:timestamp)
    n151 = local read "ThermalReadings"() -> (w327:T11[])
    n152 = local read "Pressure Reading"() -> (w319:T6)
    n153 = local read "Power Readings"() -> (w328:T10[])
    n154 = local read "Laser Readings"() -> (w325:T4)
    n155 = local read "Sensor Error 2"() -> (w316:errorcluster)
    n156 = local read "ToF Readings"() -> (w322:T7[])
    n157 = local read "Pod State Status"() -> (w324:T2)
    n158 = local read "Sensor Error"() -> (w317:errorcluster)
    n159 = local read "Laser Error"() -> (w318:errorcluster)
    n160 = local read "CPU loads"() -> (w321:T8[])
    n161 = local read "State Error"() -> (w315:errorcluster)
    n162 = local read "Actuators"() -> (w320:u32)
    n163 = Bundle(cluster=T29 {"Power Readings"=[{"Voltage (Total)"=0.0, "Bus Voltage"=0.0, "Shunt Voltage"=0.0, "Power"=0.0, "Current"=0.0, "Online"=FALSE, "Time Stamp"=timestamp(0 s since 1904-01-01)}, {"Voltage (Total)"=13.1728, "Bus Voltage"=13.148, "Shunt Voltage"=0.024800000000000003, "Power"=3.1746448000000003, "Current"=0.24100000000000002, "Online"=TRUE, "Time Stamp"=timestamp(2082864055.371957 s since 1904-01-01)}, {"Voltage (Total)"=24.13995, "Bus Voltage"=24.14, "Shunt Voltage"=-5e-05, "Power"=-0.002413995, "Current"=-0.0001, "Online"=TRUE, "Time Stamp"=timestamp(2082864055.374175 s since 1904-01-01)}], "ThermalReadings"=[{"Object Temp (°C)"=23.0625, "Object Temp (°F)"=73.5125, "Ambient Temp (°C)"=24.09375, "Ambient Temp (°F)"=75.36875, "Online"=TRUE, "Time Stamp"=timestamp(2082864055.392536 s since 1904-01-01)}, {"Object Temp (°C)"=22.84375, "Object Temp (°F)"=73.11875, "Ambient Temp (°C)"=24.0625, "Ambient Temp (°F)"=75.3125, "Online"=TRUE, "Time Stamp"=timestamp(2082864055.394416 s since 1904-01-01)}], "Analog Pressure Reading"={"HP"=-248.613281392, "MP"=-248.613281392, "LP"=-248.959961044, "BP"=-248.613281392, "Time Stamp"=timestamp(2082864055.390519 s since 1904-01-01)}, "Laser Readings"={"Fancy Laser 1"={"Laser"=FALSE, "Stripe Count"=0, "Last 10 Rising Edges"=[]}, "Fancy Laser 2"={"Laser"=FALSE, "Stripe Count"=0, "Last 10 Rising Edges"=[]}, "Simple Laser 1"={"Laser"=FALSE, "Stripe Count"=0, "Last 10 Rising Edges"=[]}, "Simple Laser 2"={"Laser"=TRUE, "Stripe Count"=0, "Last 10 Rising Edges"=[]}, "Time Stamp"=timestamp(2082864055.32697 s since 1904-01-01)}, "Pod State"=enum."Pre-flight Testing", "seconds since 1Jan1904"=timestamp(2082864055.398343 s since 1904-01-01), "ToF Readings"=[{"Distance(mm)"=51, "Online"=TRUE, "Error\nCode"=0, "Time Stamp"=timestamp(2082864055.298114 s since 1904-01-01)}, {"Distance(mm)"=12, "Online"=TRUE, "Error\nCode"=0, "Time Stamp"=timestamp(2082864055.317715 s since 1904-01-01)}, {"Distance(mm)"=9, "Online"=TRUE, "Error\nCode"=0, "Time Stamp"=timestamp(2082864055.335987 s since 1904-01-01)}, {"Distance(mm)"=25, "Online"=TRUE, "Error\nCode"=0, "Time Stamp"=timestamp(2082864055.353802 s since 1904-01-01)}], "CPU loads"=[{"Total (%)"=78.03635031413472, "Time Critical (%)"=0.0, "Timed Structures (%)"=0.32081374652993544, "High (%)"=0.0, "Above Normal (%)"=0.0, "Normal (%)"=76.33465617759227, "Background (%)"=0.0, "Idle (%)"=21.963649685865278, "ISR (%)"=1.3808803900125173}, {"Total (%)"=56.1031514616488, "Time Critical (%)"=0.0, "Timed Structures (%)"=21.009799080061946, "High (%)"=0.0, "Above Normal (%)"=0.0, "Normal (%)"=34.915435601607804, "Background (%)"=0.0, "Idle (%)"=43.8968485383512, "ISR (%)"=0.17791677997904956}], "Actuators"=14848, "Pressure Reading"={"Time Stamp"=timestamp(0 s since 1904-01-01), "Online"=FALSE, "Temperature (C)"=0.0, "Pressure (Pa)"=0.0, "Temperature (F)"=0.0}, "Laser Error"={"status"=FALSE, "code"=0, "source"=""}, "Sensor Error"={"status"=FALSE, "code"=0, "source"=""}, "Sensor Error 2"={"status"=FALSE, "code"=0, "source"=""}, "State Error"={"status"=FALSE, "code"=0, "source"=""}} ("All Data"), "Power Readings"=w328, "ThermalReadings"=w327, "Analog Pressure Reading"=w326, "Laser Readings"=w325, "Pod State"=w324, "seconds since 1Jan1904"=w323, "ToF Readings"=w322, "CPU loads"=w321, "Actuators"=w320, "Pressure Reading"=w319, "Laser Error"=w318, "Sensor Error"=w317, "Sensor Error 2"=w316, "State Error"=w315) -> (w314:T29)
    n164 = Wait (ms)(milliseconds to wait=u32 200) -> ()  [unwired: 1 out]
    n165 = shared-variable "NI-myRIO-1900-030d70ed\\Autonomous Pod Shared Variables.lvlib\\sendNcData"() -> (w310:bool, error out=w311:errorcluster)  [unwired: 1 in]
    n166 = Tick Count (ms)() -> (millisecond timer value=w309:u32)
    n167 = local read "Stop Button"() -> (w330:bool)
    n168 = feedback #4() -> (w308:u32)  [unwired: 1 in]
    n169 = feedback-in #4(w309) -> ()
    n170 = call "packageTelemetrySnapshot.vi"("Error In"=w311, "All Data"=w314, "Send Non-Critical Data"=w310) -> ("Latest Critical Telemetry"=→"Latest Critical Telemetry":T1)  [unwired: 7 in, 1 out]
    n171 = Subtract(x=w309, y=w308) -> (x-y=→"Data Snap Period":u32)
    n172 = shared-variable "NI-myRIO-1900-030d70ed\\Autonomous Pod Shared Variables.lvlib\\ResetLaserCount"() -> (w305:bool)  [unwired: 1 in, 1 out]
    n173 = shared-variable "NI-myRIO-1900-030d70ed\\Autonomous Pod Shared Variables.lvlib\\LaserDebounce"() -> (w304:u8)  [unwired: 1 in, 1 out]
    n174 = shared-variable "NI-myRIO-1900-030d70ed\\Autonomous Pod Shared Variables.lvlib\\ResetSensor"("Reset Sensors") -> ()  [unwired: 1 in, 1 out]
    n175 = local write "Reset Count"(w305) -> ()
    n176 = local write "Prior Lows"(w304) -> ()
  }
  n177 = Flush Queue(queue=w6, error in (no error)=w5) -> (queue out=w7:refnum<queue>, error out=w8:errorcluster)  [unwired: 1 out]
  n178 = Release Queue(queue=w7, error in (no error)=w8) -> ()  [unwired: 1 in, 3 out]
  n179 = flat-sequence {
    tunnel: w14 -> [w332]
    frame #0 {
      # "Shutdown Sequence"
      n180 = xnode "Digital output (1 sample) 3"("Activate Pneumatics (A/DIO10 (Pin 31))"=FALSE ("Levitation"), "error in (no error)"=w332) -> ()  [unwired: 1 out]
      n181 = local write "Stop Button"(FALSE ("Stop Button")) -> ()
      n182 = call "UDPSender.vi"("Action"=enum16{"Send", "Initialize", "Close"}."Close") -> ()  [unwired: 10 in, 1 out]
    }
  }
